vi "MapToRobotCoOrd.vi"(10 "WP Map":cluster{"X":dbl, "Y":dbl}) -> (2 "WP Robot":cluster{"X":dbl, "Y":dbl})   [LabVIEW 2014]
panel:
  # "This VI changes Waypoints from\nMap Coordinates to Robot Coordinates"
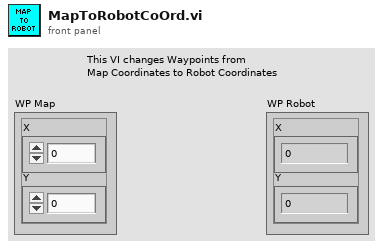
[diagram p1: front panel]
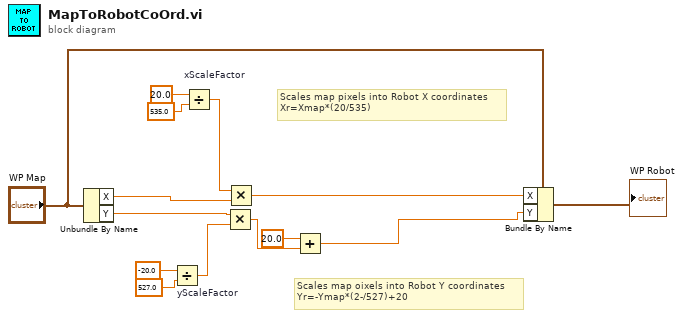
[diagram p0: block diagram]
diagram:
  # "Scales map oixels into Robot Y coordinates\nYr=-Ymap*(2-/527)+20"
  # "Scales map pixels into Robot X coordinates\nXr=Xmap*(20/535)"
  n1 = Unbundle By Name "Unbundle By Name"("WP Map") -> ("X"=w8:dbl, "Y"=w6:dbl)
  n2 = Divide "yScaleFactor"(x=-20.0, y=527.0) -> (x/y=w5:dbl)
  n3 = Divide "xScaleFactor"(x=20.0, y=535.0) -> (x/y=w7:dbl)
  n4 = Multiply(x=w6, y=w5) -> (x*y=w4:dbl)
  n5 = Multiply(x=w7, y=w8) -> (x*y=w2:dbl)
  n6 = Add(x=20.0, y=w4) -> (x+y=w1:dbl)
  n7 = Bundle By Name "Bundle By Name"(cluster="WP Map", "X"=w2, "Y"=w1) -> (→"WP Robot":cluster{"X":dbl, "Y":dbl})
